vi "Receive - UDP (CommPort).vi"() -> ()   [LabVIEW 2020]
uses:
  _controls/comm_verification_rx.ctl
  _controls/comm_udp_rx.ctl
  _polimorphicInstances/session/Fdx Create Session (Rx-VL-Oriented).vi
  bsp/AFDX_Receive/Fdx Create Rx VL.vi
  _polimorphicInstances/udpPort/Fdx Create UDP Port (RX-CommPort).vi
  _polimorphicInstances/control/Fdx Start (Rx).vi
  _polimorphicInstances/control/Fdx Stop (Rx).vi
  _polimorphicInstances/session/Fdx Close Session (Port).vi
  AIM664LV.lvlib
panel:
  out "current irig time":T1={"SignOut"=40, "DayOut"=1, "HourOut"=1, "MinOut"=28, "SecondOut"=39, "MilliSecOut"=539, "MicroSecOut"=300, "NanoSecOut"=0, "InfoOut"=0, "Mode"=3}
  in  "CommPort Config":T2={"PortType"=enum."FDX_UDP_SAMPLING", "SubVIId"=1, "domainID"=1, "sideID"=1, "locationID"=1, "partitionID"=1, "UdpSrcPort"=12345, "UdpDstPort"=12346, "UdpNumBufMessages"=0, "UdpMaxMessageSize"=1000, "UdpSamplingRate"=0} {"partitionID" format="%.0b"}
  out "BytesRead":u32
  out "Data":u8[](array[numeric])=[1, 2, 3, 4, 0, 0, 0, 0, 0, 0, 0, 0, 0, 0, 0, 0, 0, 0, 0, 0, 0, 0, 0, 0, 0, 0, 0, 0, 0, 0, 0, 0, 0, 0, 0, 0, 0, 0, 0, 0, 0, 0, 0, 0, 0, 0, 0, 0, 0, 0, 0, 0, 0, 0, 0, 0, 0, 0, 0, 0, 0, 0, 0, 0, 0, 0, 0, 0, 0, 0, 0, 0, 0, 0, 0, 0, 0, 0, 0, 0, 0, 0, 0, 0, 0, 0, 0, 0, 0, 0, 0, 0, 0, 0, 0, 0, 0, 0, 0, 0] format="%.0x"
  in  "Messages to Read (1)":u32=1
  in  "VL Config":T3={"VlId"=60, "VLRange"=2, "VerificationMode"=0, "Bag"=0, "Jitter"=0, "MaxFrameLength"=0, "MaxSkew"=0, "VLBufSize"=32768, "FilterMode"=0, "FilterPosition"=0, "Padding"=0, "FilterMask"=0, "FilterData"=0, "MinFrameLength"=0} {"FilterMode" items=["FDX_RX_VL_FLT_DIS", "FDX_RX_VL_FLT_ENA ", "FDX_RX_VL_FLT_ENA_INV"]; "MaxFrameLength" format="%.0x"; "VerificationMode" items=["FDX_RX_VL_CHECK_ENA_DEFAULT"=65535, "FDX_RX_VL_CHECK_REDMAM"=16, "DX_RX_VL_CHECK_TRAFIC"=8, "FDX_RX_VL_CHECK_FRAMESIZE"=4, "FDX_RX_VL_CHECK_SNINTEG"=2, "FDX_RX_VL_CHECK_INVPAC"=1, "FDX_RX_VL_CHECK_DISA"=0]}
  out "PortInitOut":T4={"PortConfig"=0, "PortUsed"=1, "GlobalMemFree"=0, "SharedMemFree"=0} {"PortConfig" items=["FDX_SINGLE", "FDX_REDUNDANT"]}
  in  "Port":u32=1
  in  "Board":u32
  in  "Period mS":u32=200
  out "error out":errorcluster
  in  "stop":bool
  out "current time":timestamp
  # "ARINC 664 - Receiving through UDP with Communication Port"
  # "Overview: Setup the board to transmit package as raw frames.\nRequirement: One AIM ARINC-664 board with installed AIM ARINC 664 BSP.\nRestrictions: None.\nInstruction:\n1. Select the Board ID (0 if you have only one board in your system) and the port number. If you want to validate between two ports in one device, you can use tx board and Rx Board\n2. Run the VI.\n3. See the result in Current IRIG Time"
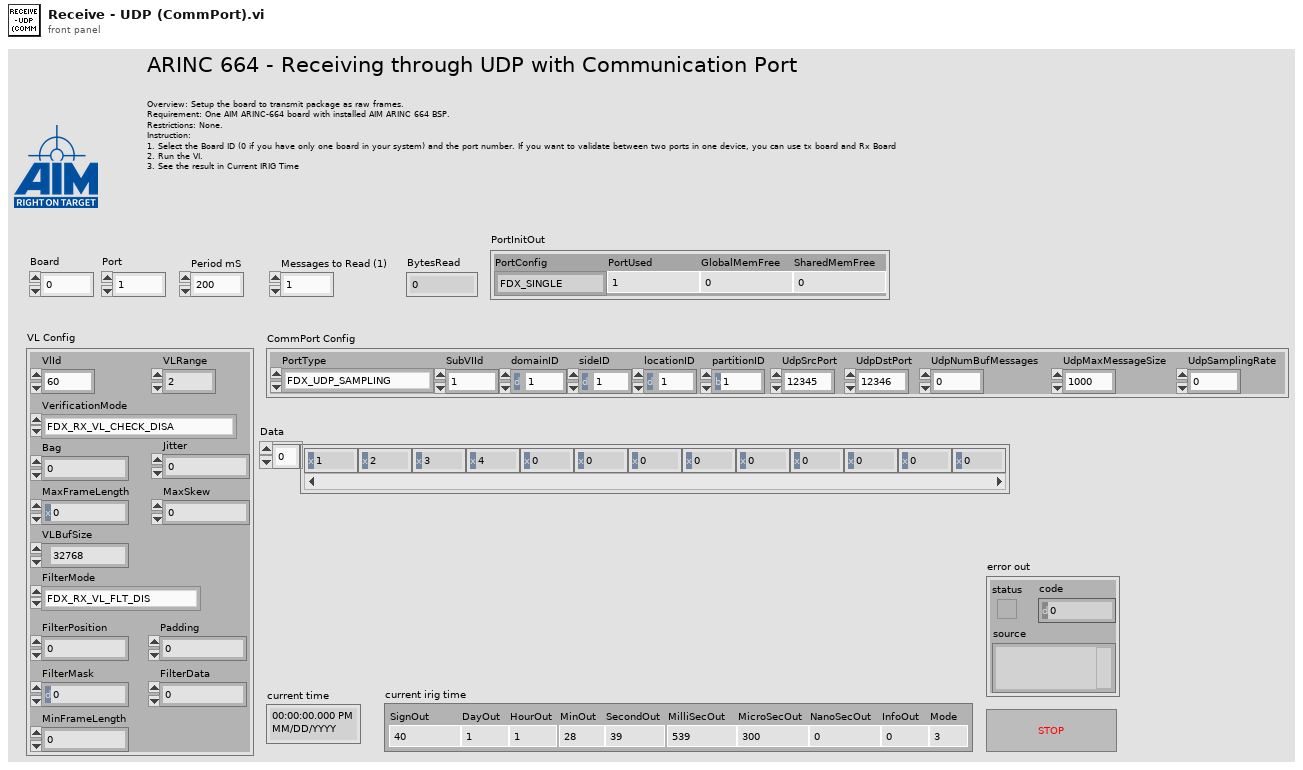
[diagram p1: front panel]
types:
  T1 = cluster{"SignOut":i32, "DayOut":u32, "HourOut":u32, "MinOut":u32, "SecondOut":u32, "MilliSecOut":u32, "MicroSecOut":u32, "NanoSecOut":u32, "InfoOut":u32, "Mode":u32}
  T2 = typedef "AIM664LV.lvlib/comm_udp_rx.ctl" = cluster{"PortType":enum16{"FDX_UDP_SAMPLING", "FDX_UDP_QUEUING"}, "SubVIId":u32, "domainID":u8, "sideID":u8, "locationID":u8, "partitionID":u8, "UdpSrcPort":u16, "UdpDstPort":u16, "UdpNumBufMessages":u32, "UdpMaxMessageSize":u32, "UdpSamplingRate":u32}
  T3 = typedef "AIM664LV.lvlib/comm_verification_rx.ctl" = cluster{"VlId":u16, "VLRange":u32, "VerificationMode":u32, "Bag":u32, "Jitter":u32, "MaxFrameLength":u32, "MaxSkew":u32, "VLBufSize":u32, "FilterMode":u32, "FilterPosition":u32, "Padding":u32, "FilterMask":u32, "FilterData":u32, "MinFrameLength":u32}
  T4 = cluster{"PortConfig":u32, "PortUsed":u32, "GlobalMemFree":u32, "SharedMemFree":u32}
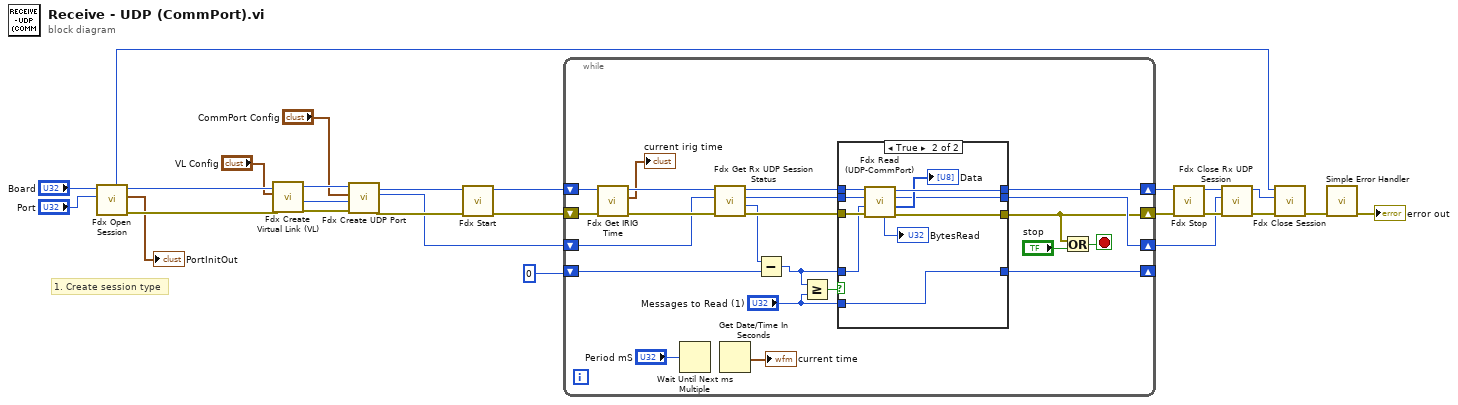
[diagram p0: block diagram]
diagram:
  # "1. Create session type"
  n1 = call-poly "Fdx Open Session.vi"("port"="Port", "board"="Board") -> ("error out"=w25:errorcluster, "PortInitOut"=→"PortInitOut":T4, "InstrumentHandle_port out"=w26:u32, "InstrumentHandle_board out"=w7:u32)  [unwired: 4 in, 2 out]
  n2 = call-poly "Fdx Create Virtual Link (VL).vi"("error in (no error)"=w25, "VL Config"="VL Config", "InstrumentHandle_port in"=w26) -> ("error out"=w23:errorcluster, "VlId"=w10:u16, "InstrumentHandle_port out"=w24:u32)  [unwired: 6 in]
  n3 = call-poly "Fdx Create UDP Port.vi"("error in"=w23, "VlId"=w10, "CommPort Config"="CommPort Config", "port handle in"=w24) -> ("error out"=w21:errorcluster, "commPort handle out"=w18:u32, "port handle out"=w22:u32)  [unwired: 4 in, 1 out]
  n4 = call-poly "Fdx Start.vi"("error in (no error)"=w21, "InstrumentHandle_port in"=w22) -> ("error out"=w4:errorcluster, "InstrumentHandle_port out"=w20:u32)  [unwired: 8 in]
  n5 = while {
    shift-right: [w41] -> w19
    shift-left: w20 -> [w37]
    shift-right: [w38] -> w5
    shift-left: w18 -> [w28]
    shift-right: [w42] -> _
    shift-left: u32 0 ("MsgCount") -> [w47]
    shift-right: [w29] -> w3
    shift-left: w4 -> [w32]
    stop <- w31 stop-if-true
    n6 = call "Fdx Get IRIG Time.vi"("error in (no error)"=w32, "InstrumentHandle_board in"=w37) -> ("error out"=w36:errorcluster, "Curent Irig Time"=→"current irig time":T1, "InstrumentHandle_board out"=w35:u32)  [unwired: 7 in]
    n7 = Wait Until Next ms Multiple(millisecond multiple="Period mS") -> ()  [unwired: 1 out]
    n8 = call "Fdx Get Rx UDP Session Status.vi"("error in (no error)"=w36, "UdpHandle in"=w28, "InstrumentHandle_port in"=w35) -> ("error out"=w46:errorcluster, "MsgCount"=w39:u32, "UdpHandle out"=w40:u32, "InstrumentHandle_port out"=w45:u32)  [unwired: 4 in, 1 out]
    n9 = Get Date/Time In Seconds() -> (seconds since 1Jan1904=→"current time":timestamp)
    n10 = Subtract(x=w39, y=w47) -> (x-y=w27:u32)
    n11 = Greater Or Equal?(x=w27, y="Messages to Read (1)") -> (x >= y?=w44:bool)
    n12 = case shown="True" w44 {
      tunnel: w46 -> [w50 w60]
      tunnel: w45 -> [w52 w61]
      tunnel: "Messages to Read (1)" -> [_ w62]
      tunnel: [w52 w59] -> w41
      tunnel: w27 -> [w51 w55]
      tunnel: [w51 w62] -> w42
      tunnel: [w50 w58] -> w29
      tunnel: w40 -> [w49 w56]
      tunnel: [w49 w53] -> w38
      frame False {
      }
      frame True {
        n13 = call "Fdx Read (UDP-CommPort).vi"("error in (no error)"=w60, "MsgCount(1)"=w55, "UdpHandle in"=w56, "InstrumentHandle_port in"=w61) -> ("error out"=w58:errorcluster, "Data"=→"Data":u8[], "UdpHandle out"=w53:u32, "InstrumentHandle_port out"=w59:u32, "MsgRead"=→"BytesRead":u32)  [unwired: 3 in]
      }
    }
    n14 = Or(x=w29, y="stop") -> (x .or. y?=w31:bool)
  }
  n15 = call-poly "Fdx Stop.vi"("error in (no error)"=w3, "InstrumentHandle_port in"=w19) -> ("error out"=w17:errorcluster, "InstrumentHandle_port out"=w6:u32)  [unwired: 8 in]
  n16 = call "Fdx Close Rx UDP Session.vi"("error in (no error)"=w17, "UdpHandle in"=w5, "InstrumentHandle_port in"=w6) -> ("error out"=w16:errorcluster, "InstrumentHandle_port out"=w8:u32)  [unwired: 7 in]
  n17 = call-poly "Fdx Close Session.vi"("error in"=w16, "InstrumentHandle_port in"=w8, "InstrumentHandle_board in"=w7) -> ("error out"=w2:errorcluster)  [unwired: 8 in]
  n18 = call <vilib>:"Simple Error Handler.vi"("error in (no error)"=w2) -> ("error out"=→"error out":errorcluster)  [unwired: 4 in, 4 out]
